vi "sub_Light.vi"(10 "Input(0-255)":u8) -> (2 "LED":u32(colorbox))   [LabVIEW 2014]
doc: "------------------------------------\nAuther: Koji Ohashi\nCopyright (c) 2020 Japan LabVIEW Users Group, Volunteer members.\nThis VI is released under the MIT License.\nhttp://opensource.org/licenses/mit-license.php\n------------------------------------"
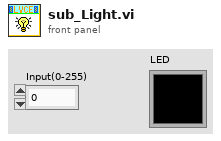
[diagram p1: front panel]
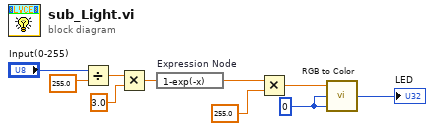
[diagram p0: block diagram]
diagram:
  w1 = u8 0 ("R")
  n1 = Divide(x="Input(0-255)", y=255.0 ("x")) -> (x/y=w4:dbl)
  n2 = Multiply(x=w4, y=3.0) -> (x*y=w3:dbl)
  n3 = expression code="1-exp(-x)"(w3) -> (w7:dbl)
  n4 = Multiply(x=w7, y=255.0) -> (x*y=w2:dbl)
  n5 = call <vilib>:"RGB to Color.vi"("B"=w1, "G"=w1, "R"=w2) -> ("Color"=→"LED":u32)
